vi "Logging ID Name Cache.vi"(1 "Name":string, 2 "ID":u32) -> (0 "ID/Name":cluster{"ID":u32, "Name":string})   [LabVIEW 2012, in "femtoRoboLib.lvlib"]
uses:
  femtoRoboLib.lvlib
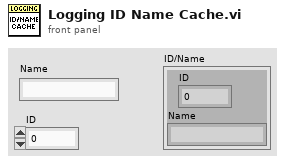
[diagram p1: front panel]
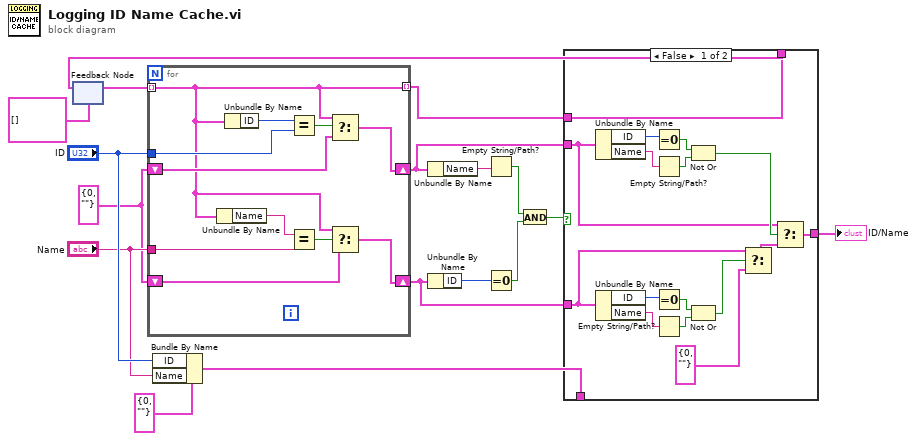
[diagram p0: block diagram]
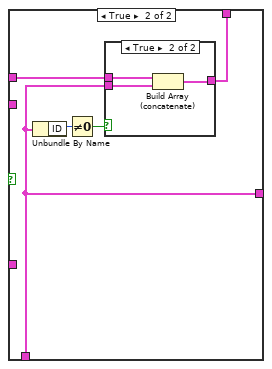
[diagram p2: hidden frame]
diagram:
  w3 = cluster{"ID":u32, "Name":string} {"ID"=0, "Name"=""} ("Written Block")
  n1 = feedback #1(cluster{"ID":u32, "Name":string}[] []) -> (w16:cluster{"ID":u32, "Name":string}[])
  n2 = for {
    tunnel: w16 -> [w18] mode=indexing
    tunnel: [w18] -> w12 mode=indexing
    shift-right: [w23] -> w7
    shift-left: w3 -> [w22]
    shift-right: [w19] -> w6
    shift-left: w3 -> [w20]
    tunnel: "ID" -> [w27]
    tunnel: "Name" -> [w26]
    n3 = Unbundle By Name(w18) -> ("Name"=w28:string)
    n4 = Unbundle By Name(w18) -> ("ID"=w25:u32)
    n5 = Equal?(x=w25, y=w27) -> (x = y?=w24:bool)
    n6 = Equal?(x=w28, y=w26) -> (x = y?=w21:bool)
    n7 = Select(t=w18, s=w24, f=w22) -> (s? t:f=w23:cluster{"ID":u32, "Name":string})
    n8 = Select(t=w18, s=w21, f=w20) -> (s? t:f=w19:cluster{"ID":u32, "Name":string})
  }
  n9 = Bundle By Name(cluster=cluster{"ID":u32, "Name":string} {"ID"=0, "Name"=""} ("Written Block"), "ID"="ID", "Name"="Name") -> (w8:cluster{"ID":u32, "Name":string})
  n10 = Unbundle By Name(w7) -> ("Name"=w15:string)
  n11 = Unbundle By Name(w6) -> ("ID"=w14:u32)
  n12 = Empty String/Path?(string/path=w15) -> (empty?=w2:bool)
  n13 = Equal To 0?(x=w14) -> (x = 0?=w1:bool)
  n14 = And(x=w2, y=w1) -> (x .and. y?=w13:bool)
  n15 = case shown="False" w13 {
    tunnel: w12 -> [w44 w49]
    tunnel: w8 -> [_ w46]
    tunnel: w7 -> [w34 _]
    tunnel: w6 -> [w31 _]
    tunnel: [w29 w46] -> w5
    tunnel: [w44 w48] -> w4
    frame False {
      n16 = Unbundle By Name(w34) -> ("ID"=w43:u32, "Name"=w42:string)
      n17 = Unbundle By Name(w31) -> ("ID"=w37:u32, "Name"=w36:string)
      n18 = Equal To 0?(x=w43) -> (x = 0?=w41:bool)
      n19 = Empty String/Path?(string/path=w42) -> (empty?=w40:bool)
      n20 = Equal To 0?(x=w37) -> (x = 0?=w38:bool)
      n21 = Empty String/Path?(string/path=w36) -> (empty?=w39:bool)
      n22 = Not Or(1:w40, 2:w41) -> (0:w35:bool)
      n23 = Not Or(1:w39, 2:w38) -> (0:w32:bool)
      n24 = Select(t=w31, s=w32, f=cluster{"ID":u32, "Name":string} {"ID"=0, "Name"=""}) -> (s? t:f=w33:cluster{"ID":u32, "Name":string})
      n25 = Select(t=w34, s=w35, f=w33) -> (s? t:f=w29:cluster{"ID":u32, "Name":string})
    }
    frame True {
      n26 = Unbundle By Name(w46) -> ("ID"=w45:u32)
      n27 = Not Equal To 0?(x=w45) -> (x != 0?=w47:bool)
      n28 = case shown="True" w47 {
        tunnel: w49 -> [w50 w53]
        tunnel: w46 -> [_ w52]
        tunnel: [w50 w51] -> w48
        frame False {
        }
        frame True {
          n29 = Build Array (concatenate)(w53, w52) -> (w51:cluster{"ID":u32, "Name":string}[])
        }
      }
    }
  }
  "ID/Name" <- w5
  n30 = feedback-in #1(w4) -> ()
